vi "Rename Close Reference VIs.vi"   [LabVIEW 2015]
uses:
  Project Manipulation Scripts/Project Manipulation Scripts.lvlib
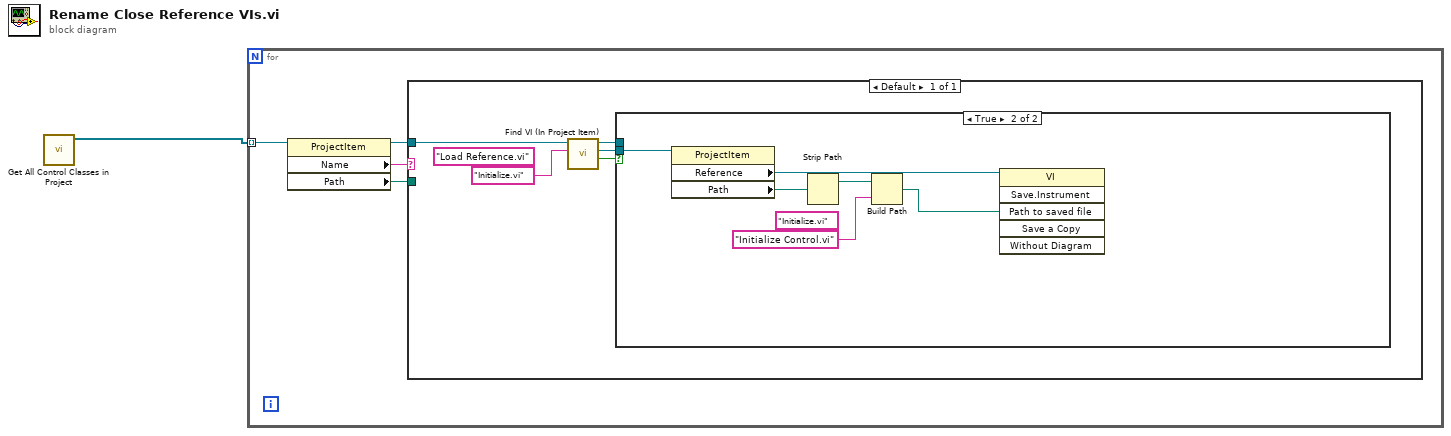
[diagram p0: block diagram]
diagram:
  n1 = call "Get All Control Classes in Project.vi"() -> ("All Control Classes"=w1:refnum<vi>[])  [unwired: 11 in]
  n2 = for {
    tunnel: w1 -> [w5] mode=indexing
    n3 = property class="ProjectItem"(reference=w5) -> (reference out=w3:refnum<vi>, "Name"=w4:string, "Path"=w2:path)  [unwired: 1 in, 1 out]
    n4 = case shown="Default" w4 {
      tunnel: w3 -> [w10]
      tunnel: w2 -> [_]
      frame Default {
        (unwired) "Load Reference.vi" ("format string")
        n5 = call "Find VI (In Project Item).vi"("VI Name"="Initialize.vi" ("name or relative path"), "ProjectItem in"=w10) -> ("Found?"=w8:bool, "VI ProjectItem Refnum"=w9:refnum<vi>, "ProjectItem out"=w7:refnum<vi>)  [unwired: 7 in]
        n6 = case shown="True" w8 {
          tunnel: w9 -> [_ w16]
          tunnel: w7 -> [_ _]
          frame False {
          }
          frame True {
            (unwired) "Initialize.vi" ("name or relative path")
            n7 = property class="ProjectItem"(reference=w16) -> ("Reference"=w15:refnum<vi>, "Path"=w14:path)  [unwired: 1 in, 2 out]
            n8 = Strip Path(path=w14) -> (stripped path=w13:path)  [unwired: 1 out]
            n9 = Build Path(base path=w13, name or relative path="Initialize Control.vi" ("format string")) -> (appended path=w12:path)
            n10 = invoke class="VI" method="Save.Instrument"(reference=w15, "Path to saved file"=w12) -> ()  [unwired: 4 in, 6 out]
          }
        }
      }
    }
  }
